vi "mass_center.vi"(11 "coordinates":dbl[][](array[numeric])) -> (0 "mass center":dbl[](array[numeric]))   [LabVIEW 2017]
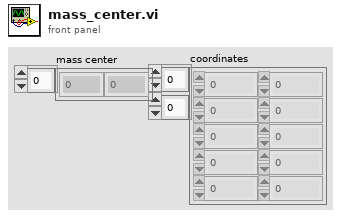
[diagram p1: front panel]
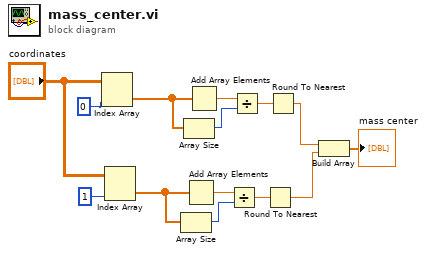
[diagram p0: block diagram]
diagram:
  n1 = Index Array(array="coordinates", index (col)=0 ("index (row)")) -> (element=w11:dbl[])  [unwired: 1 in]
  n2 = Index Array(array="coordinates", index (col)=1 ("index (row)")) -> (element=w4:dbl[])  [unwired: 1 in]
  n3 = Array Size(array=w4) -> (size(s)=w6:i32)
  n4 = Array Size(array=w11) -> (size(s)=w9:i32)
  n5 = Add Array Elements(numeric array=w4) -> (sum=w5:dbl)
  n6 = Add Array Elements(numeric array=w11) -> (sum=w10:dbl)
  n7 = Divide(x=w5, y=w6) -> (x/y=w7:dbl)
  n8 = Divide(x=w10, y=w9) -> (x/y=w8:dbl)
  n9 = Round To Nearest(number=w7) -> (nearest integer value=w2:dbl)
  n10 = Round To Nearest(number=w8) -> (nearest integer value=w3:dbl)
  n11 = Build Array(w3, w2) -> (→"mass center":dbl[])
